vi "DigitaltoBinary.vi"() -> ()   [LabVIEW 2012]
panel:
  out "Array of digits":i32[](array[numeric])
  out "Binary string":dbl
  out "Waveform Graph":dynamicdata(graph)
  out "Array of voltages":dbl[](array[numeric])
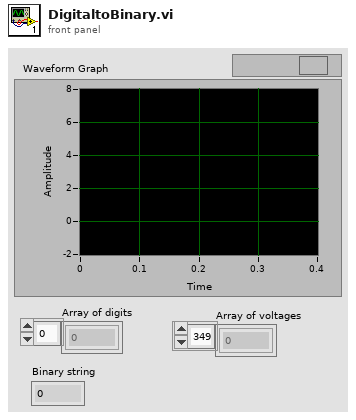
[diagram p1: front panel]
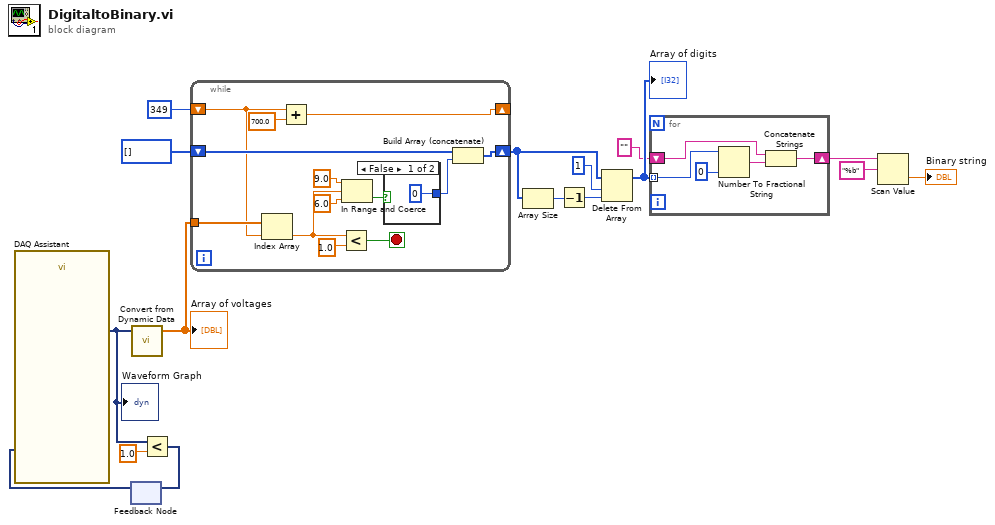
[diagram p0: block diagram]
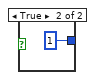
[diagram p2: hidden frame]
diagram:
  n1 = feedback #1() -> (w14:dynamicdata)  [unwired: 1 in]
  n2 = call "DAQ Assistant"("stop (T)"=w14) -> ("data"=w13:dynamicdata)  [unwired: 16 in, 2 out]
  "Waveform Graph" <- w13
  n3 = call "Convert from Dynamic Data"("Dynamic Data Type"=w13) -> ("Array"=w11:dbl[])  [unwired: 3 in]
  "Array of voltages" <- w11
  n4 = Less?(x=w13, y=1.0) -> (x < y?=w15:dynamicdata)
  n5 = feedback-in #1(w15) -> ()
  n6 = while {
    shift-right: [w19] -> _
    shift-left: 349 -> [w20]
    tunnel: w11 -> [w29]
    shift-right: [w24] -> w6
    shift-left: i32[] [] -> [w23]
    stop <- w18 stop-if-true
    n7 = Index Array(array=w29, index=w20) -> (element=w25:dbl)
    n8 = Add(x=w20, y=700.0) -> (x+y=w19:dbl)
    n9 = Less?(x=w25, y=1.0) -> (x < y?=w18:bool)
    n10 = In Range and Coerce(upper limit=9.0, x=w25, lower limit=6.0) -> (In Range?=w17:bool)  [unwired: 1 out]
    n11 = case shown="False" w17 {
      tunnel: [0 1] -> w22
      frame False {
      }
      frame True {
      }
    }
    n12 = Build Array (concatenate)(w23, w22) -> (w24:i32[])
  }
  n13 = Array Size(array=w6) -> (size(s)=w8:i32)
  n14 = Decrement(x=w8) -> (x-1=w7:i32)
  n15 = Delete From Array(array=w6, length=1, index=w7) -> (array with subset deleted=w3:i32[])  [unwired: 1 out]
  "Array of digits" <- w3
  n16 = for {
    tunnel: w3 -> [w34] mode=indexing
    shift-right: [w36] -> w1
    shift-left: "" -> [w35]
    n17 = Number To Fractional String(number=w34, precision (6)=i16 0) -> (F-format string=w32:string)  [unwired: 2 in]
    n18 = Concatenate Strings(w35, w32) -> (w36:string)
  }
  n19 = Scan Value(string=w1, format string="%b") -> (value=→"Binary string":dbl)  [unwired: 1 in, 1 out]
